vi "ByViServerInterfaceTemplate_4x4x4_Method.vi"(8 "error in (no error)":errorcluster, 11 "Interface In(KEEP)":refnum<class>) -> (0 "error out":errorcluster, 3 "Interface Out(KEEP)":refnum<class>)   [LabVIEW 2016]
panel:
  # "Place Indicators here, and remember\nto connect them to the connector pane"
  # "Place Controls here, and remember\nto connect them to the connector pane"
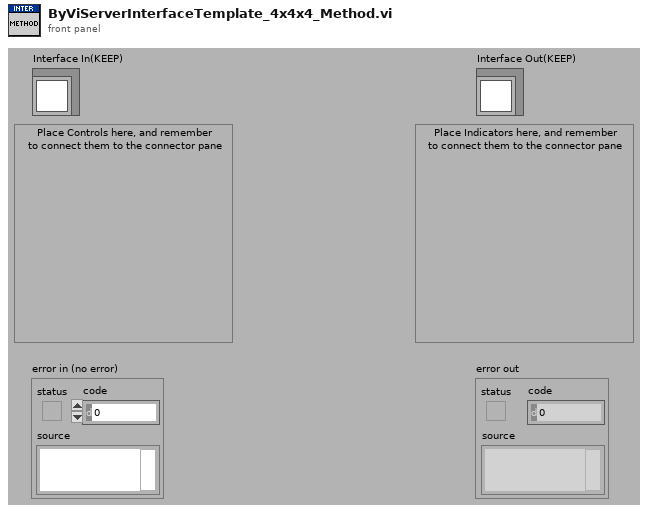
[diagram p1: front panel]
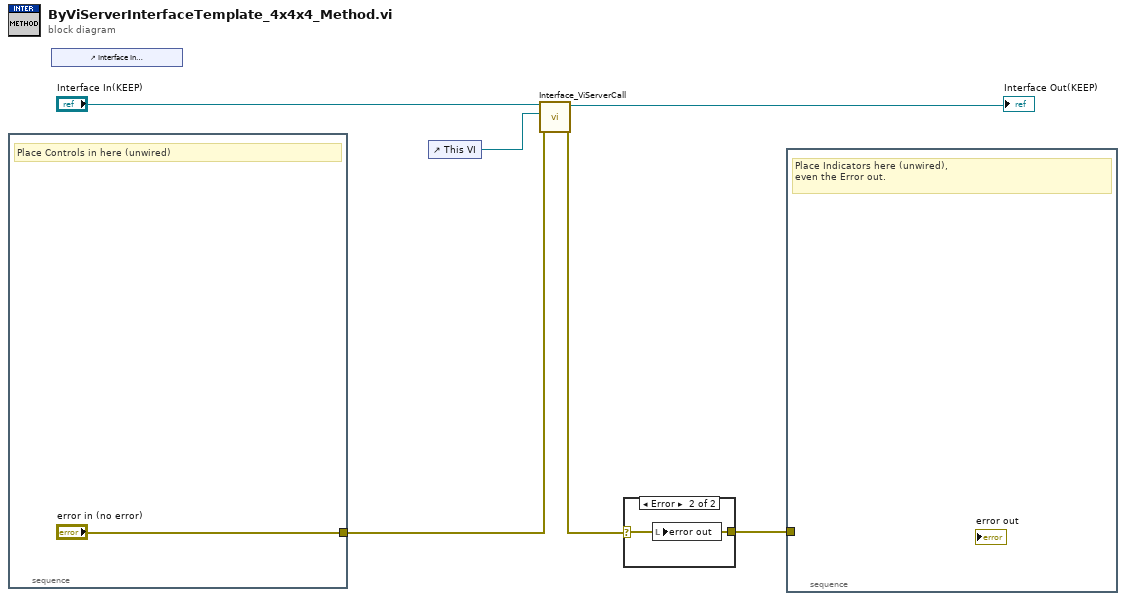
[diagram p0: block diagram]
diagram:
  n1 = stacked-sequence {
    tunnel: ["error in (no error)"] -> w4
    frame #0 {
      # "Place Controls in here (unwired)"
    }
  }
  n2 = control-ref of="Interface In\nThis reference is needed to make sure this VI's front\npanel isn't removed when building an executable."() -> ()  [unwired: 1 out]
  n3 = control-ref of="This VI"() -> (w3:refnum<vi>)
  n4 = call <vilib>:"Interface_ViServerCall.vi"("error in (no error)"=w4, "Caller VI ref (This is the interface VI's reference)"=w3, "Interface In"="Interface In(KEEP)") -> ("error out"=w2:errorcluster, "Interface Out"=→"Interface Out(KEEP)":refnum<class>)  [unwired: 7 in]
  n5 = case shown="Error" w2 {
    selector: w2 -> [w8 w9]
    tunnel: [w8 w9] -> w1
    frame No Error {
    }
    frame Error {
      n6 = local write "error out"(w9) -> ()
    }
  }
  n7 = stacked-sequence {
    tunnel: w1 -> [_]
    frame #0 {
      # "Place Indicators here (unwired),\neven the Error out."
    }
  }
